vi "Flatten.vi"(8 "error in (no error)":errorcluster, 11 "Wavelength in":refnum<class "Wavelength.lvclass">) -> (0 "error out":errorcluster, 3 "Wavelength out":refnum<class "Wavelength.lvclass">)   [LabVIEW 2017, in "Wavelength.lvclass"]
uses:
  Wavelength.lvclass
  Wavelength.lvclass/Wavelength.ctl
  Global/File Locations.vi
  Scanner/Scanner.lvclass
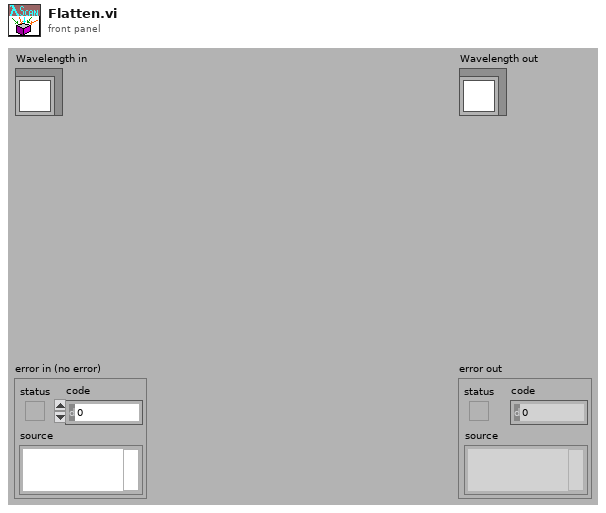
[diagram p1: front panel]
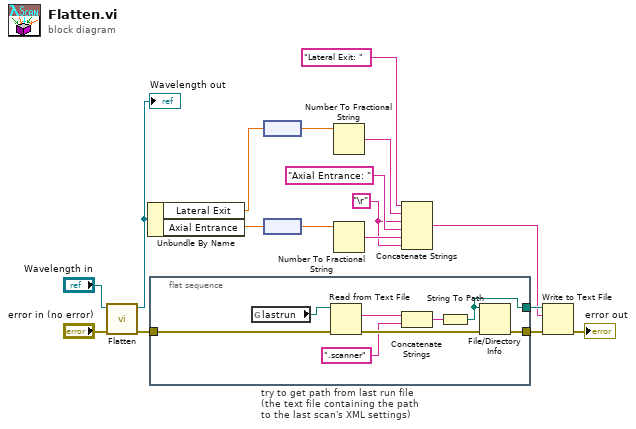
[diagram p0: block diagram]
diagram:
  w2 = "\r"
  n1 = call-parent "Flatten.vi"("error in (no error)"="error in (no error)", "Scanner in"="Wavelength in") -> ("error out"=w15:errorcluster, "Scanner out"=w11:refnum<class "Wavelength.lvclass">)  [unwired: 8 in]
  "Wavelength out" <- w11
  n2 = Unbundle By Name(w11) -> ("Lateral Exit"=w8:dbl[unit], "Axial Entrance"=w10:dbl[unit])
  n3 = flat-sequence "try to get path from last run file\n(the text file containing the path\nto the last scan's XML settings)" {
    tunnel: [w25] -> w13
    tunnel: [w22] -> w12
    tunnel: w15 -> [w21]
    frame #0 {
      n4 = global read "File Locations.vi" "lastrun"() -> (w24:path)
      n5 = Read from Text File(file (use dialog)=w24, error in=w21) -> (text=w20:string, error out=w23:errorcluster)  [unwired: 4 out]
      n6 = Concatenate Strings(w20, ".scanner") -> (w18:string)
      n7 = String To Path(string=w18) -> (path=w25:path)
      n8 = File/Directory Info(path=w25, error in=w23) -> (error out=w22:errorcluster)  [unwired: 6 out]
    }
  }
  n9 = node(w8) -> (w7:dbl)
  n10 = node(w10) -> (w9:dbl)
  n11 = Number To Fractional String(number=w7) -> (F-format string=w5:string)  [unwired: 3 in]
  n12 = Number To Fractional String(number=w9) -> (F-format string=w3:string)  [unwired: 3 in]
  n13 = Concatenate Strings("Lateral Exit: ", w5, w2, "Axial Entrance: ", w3, w2) -> (w1:string)
  n14 = Write to Text File(file (use dialog)=w13, text=w1, error in=w12) -> (error out=→"error out":errorcluster)  [unwired: 1 in, 2 out]
